vi "Render_AD_Results.vi"(4 "Background Color":u32(colorbox)=16448250, 5 "Rel._Margin":sgl=0.2, 6 "Image_Dims":cluster{"X Resolution":i32, "Y Resolution":i32}={"X Resolution"=60, "Y Resolution"=96}, 8 "error in":errorcluster, 11 "Anomaly Detection Rresults":T1={"Image"="remote image 000002063DE67978", "Ground Truth"="remote image 000002063DE67A28", "Predicted Heat Map"="remote image 000002063DE67B88", "Predicted Mask"="remote image 000002063DE699C8", "Segmentation"="remote image 000002063DE69A78"}) -> (0 "error out":errorcluster, 3 "Anomaly Detection Results":T2(plugin-control))   [LabVIEW 2020]
uses:
  PatchCore_AddOn/Low_Level/Controls/Anomaly_Detection_Results_Imgs.ctl
  <vilib>/vision/NI_Vision_Development_Module.lvlib
  PatchCore_AddOn/PatchCore_AddOn.lvlib
panel:
  out "Font Size":i16
  in  "Desired Font (Application)":T3(ring)
  in  "[User-specified Font].Font Name":string="system font"
  in  "Horizontal Alignment":i16(ring)=1 items=["Left", "Center", "Right"]
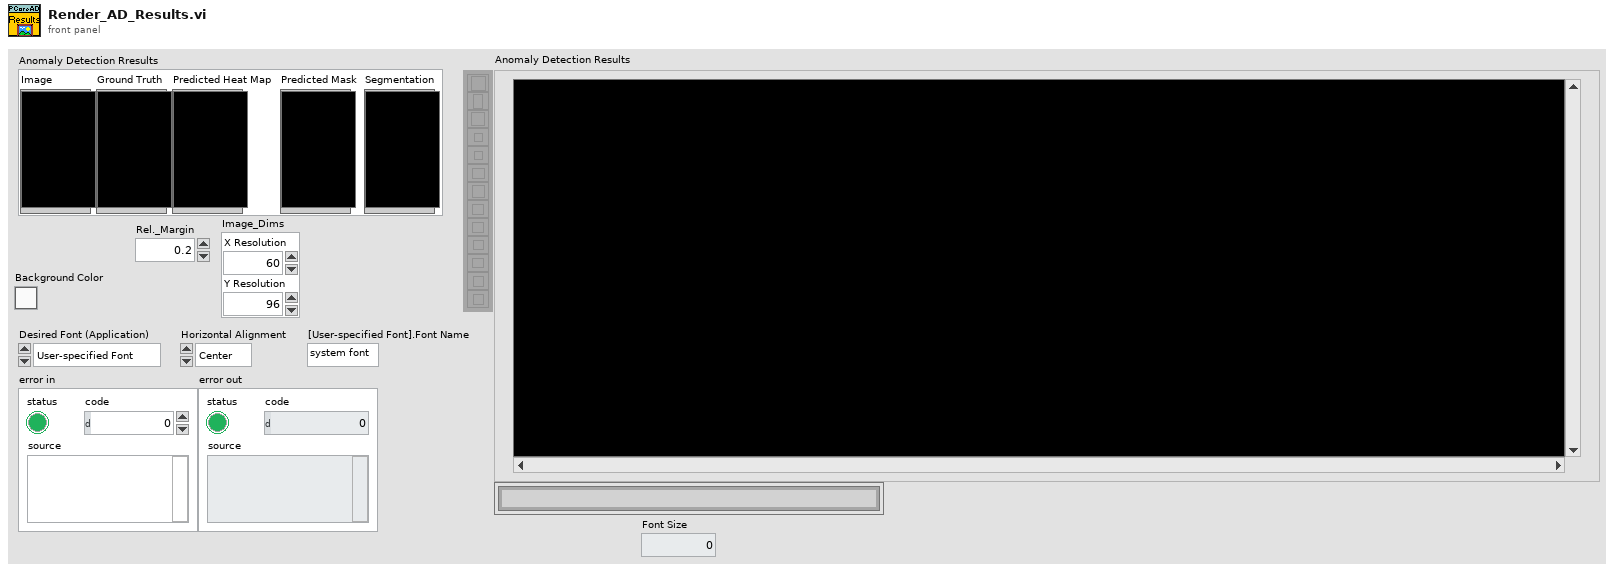
[diagram p1: front panel]
types:
  T1 = typedef "PatchCore_AddOn.lvlib/Anomaly_Detection_Results_Imgs.ctl" = cluster{"Image":T2, "Ground Truth":T2, "Predicted Heat Map":T2, "Predicted Mask":T2, "Segmentation":T2}
  T2 = typedef "IMAQ Image.ctl" = refnum<image>
  T3 = enum16{"User-specified Font", "Application Font", "System Font", "Dialog Font"}
  T4 = cluster{"Desired Font (Application)":enum16{"User-specified Font", "Application Font", "System Font", "Dialog Font"}, "[User-specified Font]":cluster{"Font Name":string, "Size":i16, "Strikeout?":bool, "Italic?":bool, "Underline?":bool, "Outline?":bool, "Shadow?":bool, "Bold?":bool, "Rotation Angle":dbl}, "Horizontal Alignment":i16, "Vertical Alignment":i16}
  T5 = typedef "Image Type" = u32
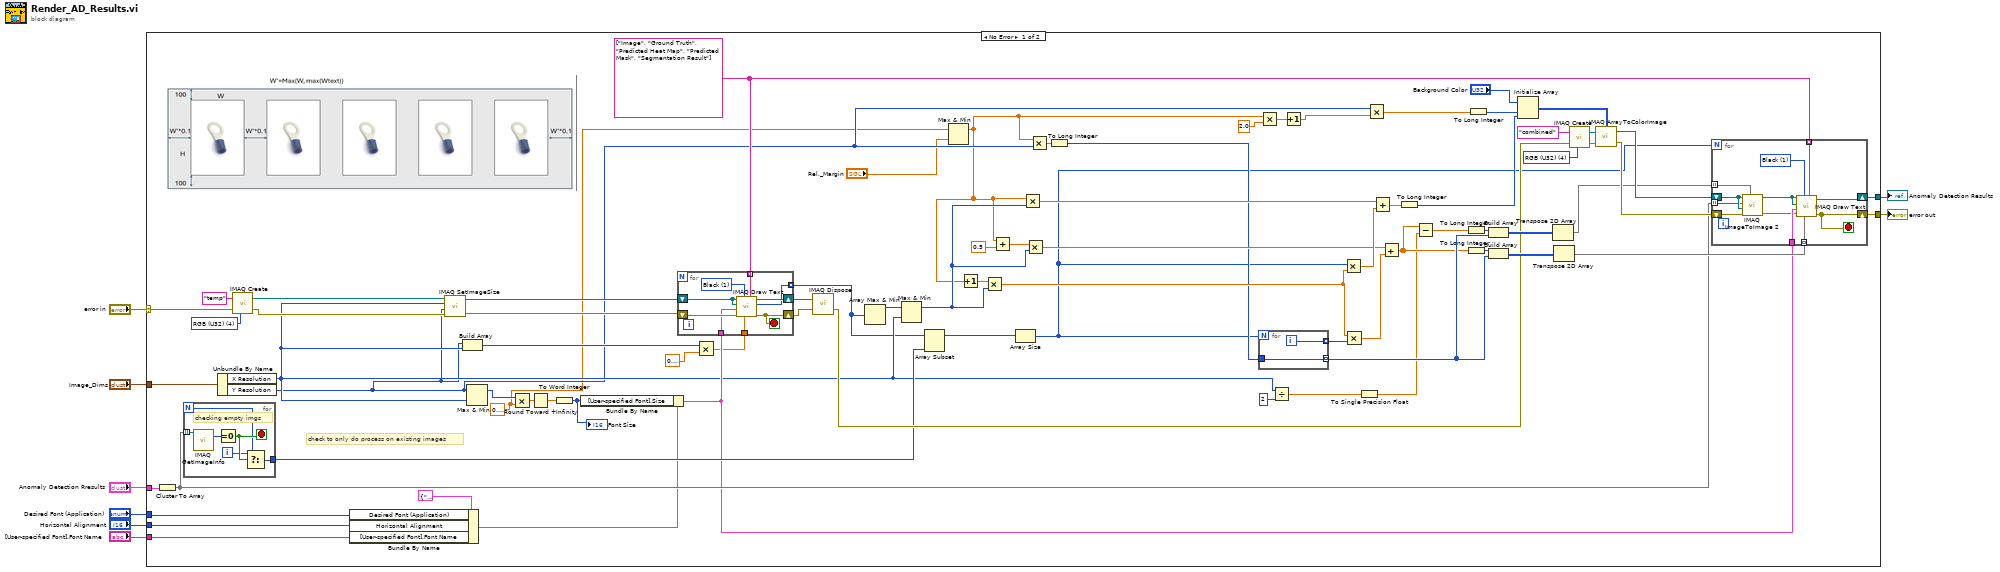
[diagram p0: block diagram]
diagram:
  n1 = case shown="No Error" "error in" {
    selector: "error in" -> [w27 w116]
    tunnel: "Horizontal Alignment" -> [w77 _]
    tunnel: "[User-specified Font].Font Name" -> [w72 _]
    tunnel: "Desired Font (Application)" -> [w71 _]
    tunnel: [w68 w116] -> w1
    tunnel: [w32 _] -> w2
    tunnel: "Image_Dims" -> [w29 _]
    tunnel: "Anomaly Detection Rresults" -> [w28 _]
    frame No Error {
      w11 = sgl 0.1 ("y")
      w36 = string[] ["Image", "Ground Truth", "Predicted Heat Map", "Predicted Mask", "Segmentation Result"] ("String")
      w43 = T5 4 items=["Grayscale (U8)", "Grayscale (I16)", "Grayscale (SGL)", "Complex (CSG)", "RGB (U32)", "HSL (U32)", "RGB (U64)", "Grayscale (U16)"] ("Image Type")
      w86 = T5 4 items=["Grayscale (U8)", "Grayscale (I16)", "Grayscale (SGL)", "Complex (CSG)", "RGB (U32)", "HSL (U32)", "RGB (U64)", "Grayscale (U16)"] ("Image Type")
      # "check to only do process on existing images"
      n2 = Cluster To Array(cluster=w28) -> (array=w25:T2[])
      n3 = for {
        N -> [w99]
        tunnel: w25 -> [w103] mode=indexing
        tunnel: [w102] -> w23
        i -> [w100]
        stop <- w101 stop-if-true
        # "checking empty imgs"
        n4 = call "IMAQ GetImageInfo"("Image"=w103) -> ("X Resolution"=w104:i32)  [unwired: 3 in, 7 out]
        n5 = Equal To 0?(x=w104) -> (x = 0?=w101:bool)
        n6 = Select(t=w100, s=w101, f=w99) -> (s? t:f=w102:i32)
      }
      n7 = Unbundle By Name(w29) -> ("X Resolution"=w18:i32, "Y Resolution"=w14:i32)
      n8 = call "IMAQ Create"("Image Name"="temp", "Image Type"=w43, "error in (no error)"=w27) -> ("New Image"=w41:T2, "error out"=w38:errorcluster)  [unwired: 2 in]
      n9 = Bundle By Name(cluster=T4 {"Desired Font (Application)"=enum."Application Font", "[User-specified Font]"={"Font Name"="", "Size"=12, "Strikeout?"=FALSE, "Italic?"=FALSE, "Underline?"=FALSE, "Outline?"=FALSE, "Shadow?"=FALSE, "Bold?"=FALSE, "Rotation Angle"=0.0}, "Horizontal Alignment"=0, "Vertical Alignment"=0} ("Font, Size & Style"), "Desired Font (Application)"=w71, "Horizontal Alignment"=w77, "[User-specified Font].Font Name"=w72) -> (w21:T4)
      n10 = call "IMAQ SetImageSize"("error in (no error)"=w38, "Y Resolution"=w14, "X Resolution"=w18, "Image"=w41) -> ("error out"=w37:errorcluster, "Image Out"=w17:T2)  [unwired: 1 in]
      n11 = Build Array(w14, w18) -> (w35:i32[])
      n12 = Max & Min(x=w14, y=w18) -> (max(x,y)=w31:i32)  [unwired: 1 out]
      n13 = Multiply(x=w31, y=w11) -> (x*y=w30:sgl)
      n14 = Round Toward +Infinity(x=w30) -> (ceil(x): smallest int >= x=w15:sgl)
      n15 = To Word Integer(number=w15) -> (16bit integer=w9:i16)
      "Font Size" <- w9
      n16 = Bundle By Name(cluster=w21, "[User-specified Font].Size"=w9) -> (w20:T4)
      n17 = Multiply(x=w35, y=sgl 0.1) -> (x*y=w19:sgl[])
      n18 = for {
        shift-right: [w114] -> w40
        shift-left: w17 -> [w110]
        tunnel: w36 -> [w113] mode=indexing
        shift-right: [w111] -> w39
        shift-left: w37 -> [w112]
        tunnel: [w109] -> w16 mode=indexing
        tunnel: w20 -> [w107]
        tunnel: w19 -> [w108]
        stop <- w111 stop-if-true
        w115 = 1 items=["White", "Black", "Inverted", "Black on White", "White on Black"] ("Color")
        n19 = call "IMAQ Draw Text"("String"=w113, "Insertion Point"=w108, "Color"=w115, "error in (no error)"=w112, "Font, Size & Style"=w107, "Image Dst"=w110, "Image Src"=w110) -> ("error out"=w111:errorcluster, "String width"=w109:i32, "Image Dst Out"=w114:T2)  [unwired: 1 in, 1 out]
      }
      n20 = call "IMAQ Dispose"("Image"=w40, "error in (no error)"=w39) -> ("error out"=w26:errorcluster)  [unwired: 4 in]
      n21 = Array Max & Min(array=w16) -> (max value=w81:i32)  [unwired: 3 out]
      n22 = Max & Min(x=w81, y=w18) -> (max(x,y)=w53:i32)  [unwired: 1 out]
      n23 = Array Subset(array=w16, length=w23) -> (w24:i32[])  [unwired: 1 in]
      n24 = Max & Min(x=w11, y="Rel._Margin") -> (max(x,y)=w10:sgl)  [unwired: 1 out]
      n25 = Increment(x=w10) -> (x+1=w58:sgl)
      n26 = Multiply(x=w58, y=w53) -> (x*y=w56:sgl)
      n27 = Add(x=w10, y=sgl 0.5) -> (x+y=w54:sgl)
      n28 = Array Size(array=w24) -> (size(s)=w22:i32)
      n29 = Multiply(x=w10, y=w53) -> (x*y=w57:sgl)
      n30 = Multiply(x=w54, y=w53) -> (x*y=w52:sgl)
      n31 = Multiply(x=w10, y=w14) -> (x*y=w13:sgl)
      n32 = To Long Integer(number=w13) -> (32bit integer=w44:i32)
      n33 = for {
        N: w22 -> [_]
        tunnel: [w106] -> w66 mode=indexing
        tunnel: [w105] -> w64 mode=indexing
        tunnel: w44 -> [w105]
        i -> [w106]
      }
      n34 = Multiply(x=w10, y=sgl 2.0) -> (x*y=w75:sgl)
      n35 = Divide(x=w18, y=2) -> (x/y=w62:dbl)
      n36 = Increment(x=w75) -> (x+1=w46:sgl)
      n37 = Multiply(x=w22, y=w56) -> (x*y=w60:sgl)
      n38 = Multiply(x=w56, y=w66) -> (x*y=w65:sgl[])
      n39 = To Single Precision Float(number=w62) -> (single precision float=w47:sgl)
      n40 = Multiply(x=w14, y=w46) -> (x*y=w73:sgl)
      n41 = Add(x=w57, y=w60) -> (x+y=w67:sgl)
      n42 = Add(x=w52, y=w65) -> (x+y=w63:sgl[])
      n43 = To Long Integer(number=w67) -> (32bit integer=w59:i32)
      n44 = Subtract(x=w63, y=w47) -> (x-y=w61:sgl[])
      n45 = To Long Integer(number=w61) -> (32bit integer=w48:i32[])
      n46 = To Long Integer(number=w63) -> (32bit integer=w49:i32[])
      n47 = To Long Integer(number=w73) -> (32bit integer=w45:i32)
      n48 = Build Array(w48, w64) -> (w80:i32[][])
      n49 = Build Array(w49, w64) -> (w79:i32[][])
      n50 = Initialize Array("Background Color", w45, w59) -> (w84:u32[][])
      n51 = Transpose 2D Array(2D array=w80) -> (transposed array=w51:i32[][])
      n52 = Transpose 2D Array(2D array=w79) -> (transposed array=w50:i32[][])
      n53 = call "IMAQ Create"("Image Name"="combined", "Image Type"=w86, "error in (no error)"=w26) -> ("New Image"=w83:T2, "error out"=w70:errorcluster)  [unwired: 2 in]
      n54 = call "IMAQ ArrayToColorImage"("Image Pixels (U32)"=w84, "Image"=w83, "error in (no error)"=w70) -> ("Image Out"=w82:T2, "error out"=w69:errorcluster)  [unwired: 2 in]
      n55 = for {
        N: w22 -> [_]
        tunnel: w25 -> [w91] mode=indexing
        shift-right: [w97] -> w32
        shift-left: w82 -> [w92]
        tunnel: w36 -> [w96] mode=indexing
        tunnel: w51 -> [w95] mode=indexing
        tunnel: w50 -> [w94] mode=indexing
        tunnel: w20 -> [w93]
        shift-right: [w87] -> w68
        shift-left: w69 -> [w90]
        stop <- w87 stop-if-true
        w98 = 1 items=["White", "Black", "Inverted", "Black on White", "White on Black"] ("Color")
        n56 = call "IMAQ ImageToImage 2"("Offset Left/Top"=w95, "error in (no error)"=w90, "Image Dst"=w92, "Image Src (Small)"=w91, "Image Src (Large)"=w92) -> ("error out"=w89:errorcluster, "Image Dst Out"=w88:T2)  [unwired: 5 in]
        n57 = call "IMAQ Draw Text"("String"=w96, "Insertion Point"=w94, "Color"=w98, "error in (no error)"=w89, "Font, Size & Style"=w93, "Image Dst"=w88, "Image Src"=w88) -> ("error out"=w87:errorcluster, "Image Dst Out"=w97:T2)  [unwired: 1 in, 2 out]
      }
    }
    frame Error {
    }
  }
  "Anomaly Detection Results" <- w2
  "error out" <- w1
